vi "Simple_DAQ_AnalogIO.set voltage.vi"(0 "i ref in":refnum<vi>, 3 "Timeout":i32=10000, 5 "error in":errorcluster caption="Fehler (Eingang, kein Fehler)", 9 "voltage":dbl) -> (14 "i ref out":refnum<vi>, 17 "timed out":bool, 19 "error out":errorcluster caption="Fehler (Ausgang)")   [LabVIEW 2014, in "Simple_DAQ_AnalogIO.lvlib"]
doc: "Contact: Falk Ziegler, eMail: info@lab-coding.de"
uses:
  Simple_DAQ_AnalogIO.lvlib
  CS_Core/CSApplicationBaseClasses/PSChannelBase/PSChannelBase.lvlib
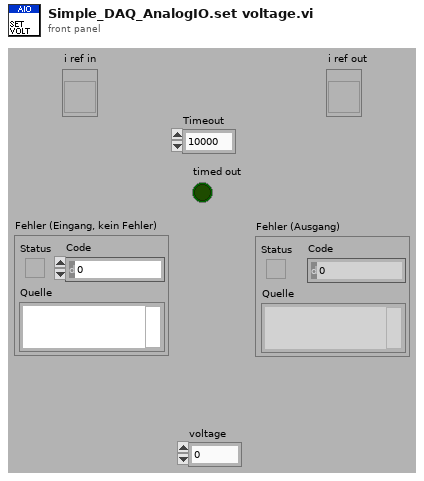
[diagram p1: front panel]
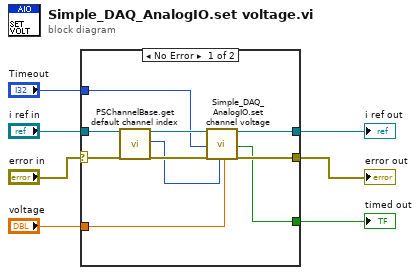
[diagram p0: block diagram]
diagram:
  n1 = case shown="No Error" "error in" {
    selector: "error in" -> [w16 w18]
    tunnel: "i ref in" -> [w17 w19]
    tunnel: [w9 w19] -> w5
    tunnel: "Timeout" -> [w12 _]
    tunnel: "voltage" -> [w13 _]
    tunnel: [w10 w18] -> w2
    tunnel: [w8 _] -> w1
    frame No Error {
      n2 = call "PSChannelBase.get default channel index.vi"("i ref in"=w17, "error in (no error)"=w16) -> ("i ref out"=w14:refnum<vi>, "defaultChannelIndex"=w11:i32, "error out"=w15:errorcluster)  [unwired: 15 in]
      n3 = call "Simple_DAQ_AnalogIO.set channel voltage.vi"("i ref in"=w14, "Timeout"=w12, "error in"=w15, "channel_index"=w11, "voltage"=w13) -> ("i ref out"=w9:refnum<vi>, "timed out"=w8:bool, "error out"=w10:errorcluster)  [unwired: 12 in]
    }
    frame Error {
    }
  }
  "error out" <- w2
  "timed out" <- w1
  "i ref out" <- w5
